vi "Write SensorInfo.vi"(8 "error in (no error)":errorcluster, 10 "Sensor Definition.lvlib:SensorInfo.lvclass":refnum<class "SensorInfo.lvclass">, 11 "SensorCharm in":refnum<class "SensorCharm.lvclass">) -> (0 "error out":errorcluster, 3 "SensorCharm out":refnum<class "SensorCharm.lvclass">)   [LabVIEW 2012, in "Sensor Definition.lvlib" / "SensorCharm.lvclass"]
uses:
  SensorCharm.lvclass
  SensorInfo.lvclass
  SensorCharm.lvclass/SensorCharm.ctl
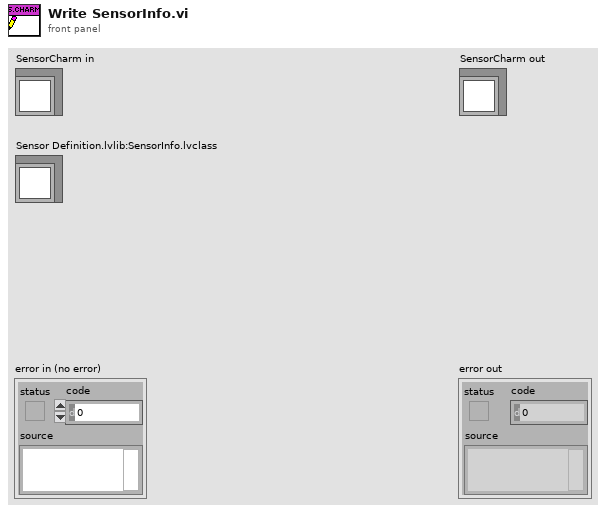
[diagram p1: front panel]
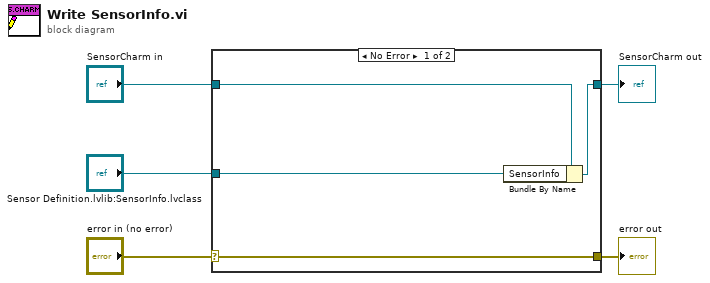
[diagram p0: block diagram]
diagram:
  n1 = case shown="No Error" "error in (no error)" {
    selector: "error in (no error)" -> [w9 w10]
    tunnel: [w9 w10] -> w4
    tunnel: [w7 w11] -> w2
    tunnel: "SensorCharm in" -> [w8 w11]
    tunnel: "Sensor Definition.lvlib:SensorInfo.lvclass" -> [w6 _]
    frame No Error {
      n2 = Bundle By Name(cluster=w8, "SensorInfo"=w6) -> (w7:refnum<class "SensorCharm.lvclass">)
    }
    frame Error {
    }
  }
  "error out" <- w4
  "SensorCharm out" <- w2
